vi "test.RegisterModule.vi"() -> ()   [LabVIEW 2014]
uses:
  Private/Class/meth.Constructor.vi
  Private/Class/meth.Destructor.vi
  GLue.lvlib
panel:
  out "Return Data":variant
  out "error out":errorcluster
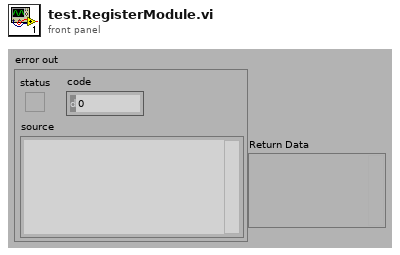
[diagram p1: front panel]
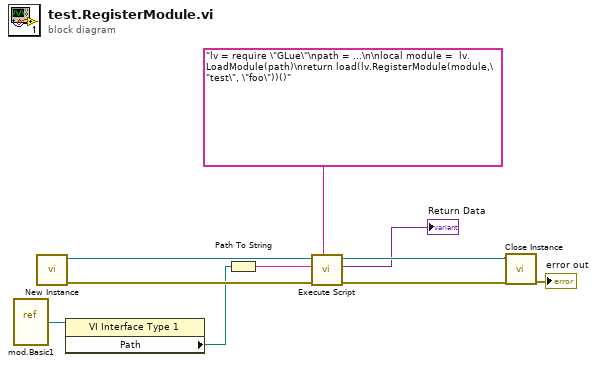
[diagram p0: block diagram]
diagram:
  n1 = vi-ref "mod.Basic1.vi"() -> (w4:refnum<vi>)
  n2 = call "New Instance.vi"() -> ("error out"=w5:errorcluster, "GLue out"=w6:refnum<class "class.GLue.lvclass">)  [unwired: 10 in]
  n3 = property class="VI Interface Type 1"(reference=w4) -> ("Path"=w2:path)  [unwired: 1 in, 2 out]
  n4 = Path To String(path=w2) -> (string=w1:string)
  n5 = call "Execute Script.vi"("Script"="lv = require \"GLue\"\npath = ...\n\nlocal module =  lv.LoadModule(path)\nreturn load(lv.RegisterModule(module,\"test\", \"foo\"))()", "error in"=w5, "Argument Data"=w1, "GLue in"=w6) -> ("error out"=w8:errorcluster, "Return Data"=→"Return Data":variant, "GLue out"=w7:refnum<class "class.GLue.lvclass">)  [unwired: 5 in]
  n6 = call "Close Instance.vi"("error in"=w8, "GLue in"=w7) -> ("error out"=→"error out":errorcluster)  [unwired: 9 in]
